vi "FTW-Regex-Construct.vi"(5 "Regular Expression":string, 11 "error in":errorcluster) -> (4 "Regex":refnum<class "FTW-Regex.lvclass">, 15 "error out":errorcluster)   [LabVIEW 2014, in "FTW-Regex.lvclass"]
uses:
  FTW-Regex.lvclass
  FTW-Regex.lvclass/FTW-Regex.ctl
  error/FTW-ERR-ThrowError.vi
  error/FTW-ERR-NoErrorConstant.vi
  error/FTW-ERR-CallChain.vi
  string/FTW-STR-ReplaceWhitespace.vi
panel:
  # "Inputs"
  # "Outputs"
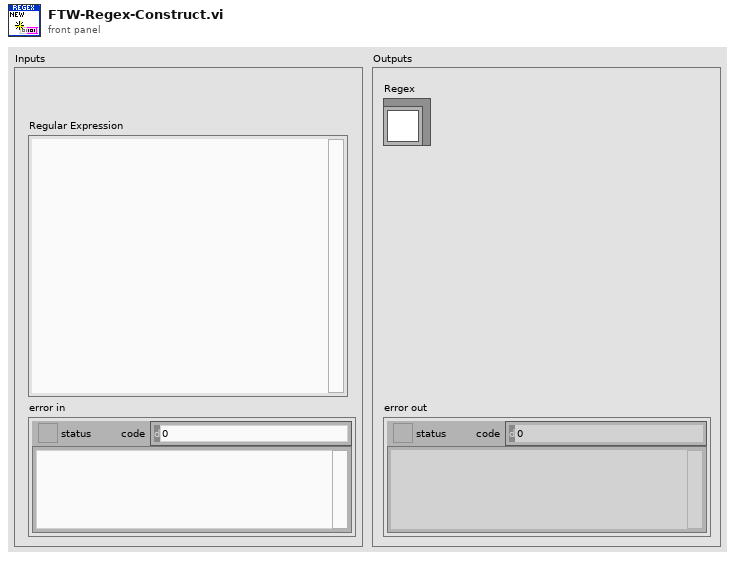
[diagram p1: front panel]
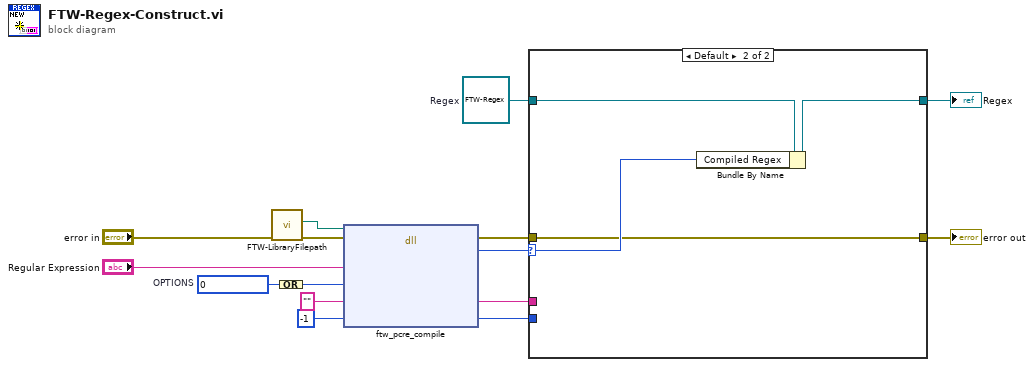
[diagram p0: block diagram]
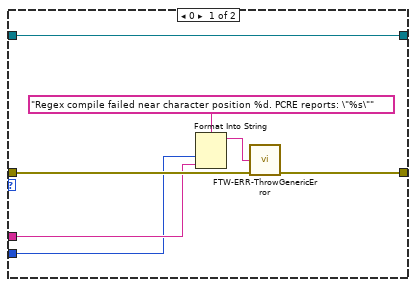
[diagram p2: hidden frame]
diagram:
  w10 = 0  # OPTIONS
  w6 = refnum<class "FTW-Regex.lvclass"> refnum  # Regex
  n1 = call "FTW-LibraryFilepath.vi"("error in"="error in") -> ("error out"=w14:errorcluster, "Library Filepath"=w15:path)  [unwired: 8 in, 1 out]
  n2 = Compound Arithmetic op=OR(w10) -> (w11:i32)
  n3 = dll-call lib="?" fn="ftw_pcre_compile"(path in=w15, error in=w14, "Pattern"="Regular Expression", "Options"=w11, "Error String"="", "Error Offset in Pattern"=i64 -1) -> (error out=w5:errorcluster, "Compiled Regex"=w8:u64, "Error String"=w3:string, "Error Offset in Pattern"=w1:i64)  [unwired: 3 in, 1 out]
  n4 = case shown="Default" w8 {
    selector: w8 -> [_ w24]
    tunnel: [w22 w25] -> w7
    tunnel: w6 -> [w22 w26]
    tunnel: w5 -> [w21 w23]
    tunnel: [w20 w23] -> w4
    tunnel: w3 -> [w17 _]
    tunnel: w1 -> [w16 _]
    frame 0 {
      n5 = Format Into String(format string="Regex compile failed near character position %d. PCRE reports: \"%s\"", w16, w17) -> (resulting string=w19:string)  [unwired: 2 in, 1 out]
      n6 = call "FTW-ERR-ThrowGenericError.vi"("Error Message"=w19, "error in"=w21) -> ("error out"=w20:errorcluster)  [unwired: 13 in]
    }
    frame Default {
      n7 = Bundle By Name(cluster=w26, "Compiled Regex"=w24) -> (w25:refnum<class "FTW-Regex.lvclass">)
    }
  }
  "error out" <- w4
  "Regex" <- w7
